vi "Assert To Report Entry.vi"(8 "error in (no error)":errorcluster, 10 "Assert":T1) -> (0 "error out":errorcluster, 2 "String":string)   [LabVIEW 2013, in "Caraya.lvlib" / "Test Report.JUnit.lvclass"]
uses:
  Test Report.JUnit.lvclass
  Test Result/Assert Event Data.ctl
  Test Report/Test Report.lvclass
  Test Result/Test Result.lvclass
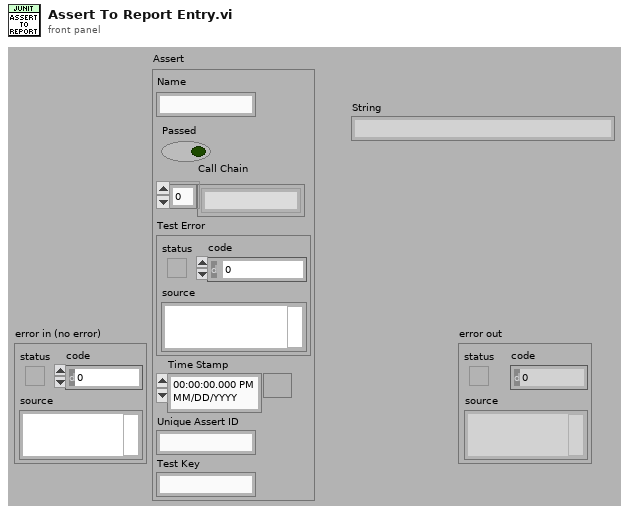
[diagram p1: front panel]
types:
  T1 = typedef "Caraya.lvlib/Test Result.lvclass/Assert Event Data.ctl" = cluster{"Name":string, "Passed":bool, "Call Chain":string[], "Test Error":errorcluster, "Time Stamp":timestamp, "Unique Assert ID":string, "Test Key":string}
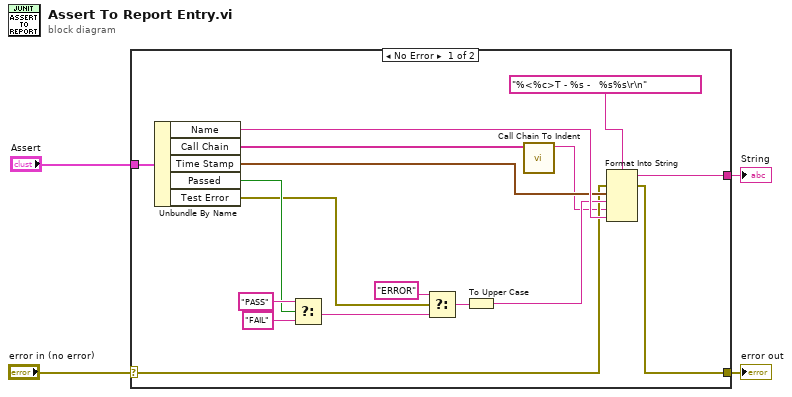
[diagram p0: block diagram]
diagram:
  n1 = case shown="No Error" "error in (no error)" {
    selector: "error in (no error)" -> [w11 w22]
    tunnel: [w19 w22] -> w3
    tunnel: "Assert" -> [w17 _]
    tunnel: [w18 _] -> w1
    frame No Error {
      n2 = Unbundle By Name(w17) -> ("Name"=w20:string, "Call Chain"=w6:string[], "Time Stamp"=w16:timestamp, "Passed"=w8:bool, "Test Error"=w7:errorcluster)
      n3 = Select(t="PASS" ("format string"), s=w8, f="FAIL" ("format string")) -> (s? t:f=w10:string)
      n4 = Select(t="ERROR" ("format string"), s=w7, f=w10) -> (s? t:f=w13:string)
      n5 = To Upper Case(1:w13) -> (0:w12:string)
      n6 = call "Call Chain To Indent.vi"("Call Chain"=w6) -> ("Indent"=w5:string)  [unwired: 10 in]
      n7 = Format Into String(format string="%<%c>T - %s -   %s%s\r\n", error in=w11, w16, w12, w5, w20) -> (resulting string=w18:string, error out=w19:errorcluster)  [unwired: 1 in]
    }
    frame Error {
    }
  }
  "error out" <- w3
  "String" <- w1
